vi "TcA02-009_TimeoutWhenWaitingForModifyingAttributes.vi"(1 "Input buffer":T3="1", 3 "Invocation info":T2, 5 "error in (no error)":errorcluster, 6 "Add log to result?":bool) -> (16 "Test Data":T1 {"Numeric Measurement" format="%.2f"}, 19 "error out":errorcluster)   [LabVIEW 2020]
doc: "Test case template."
uses:
  Shared/Support_InputBuffer.ctl
  Shared/Support_InvocationInfo.ctl
  Shared/Support_TestData.ctl
  TestClasses/G#BaseClass2_class/G#BaseClass2.lvclass
  TestClasses/G#SubClass2_class/G#SubClass2.lvclass
  TestClasses/G#SubSubClass2_class/G#SubSubClass2.lvclass
  <vilib>/addons/_AddQ/G#Object/G#Object.lvclass
panel:
  in  "Test name":string="TcA02-009 Timeout when waiting for modifying attributes"
  out "Test result":bool
  out "Result":string
  # "Verify that waiting for modifying objects attributes\nwhen mutual excluded can be timeout."
  # "Sub test case"
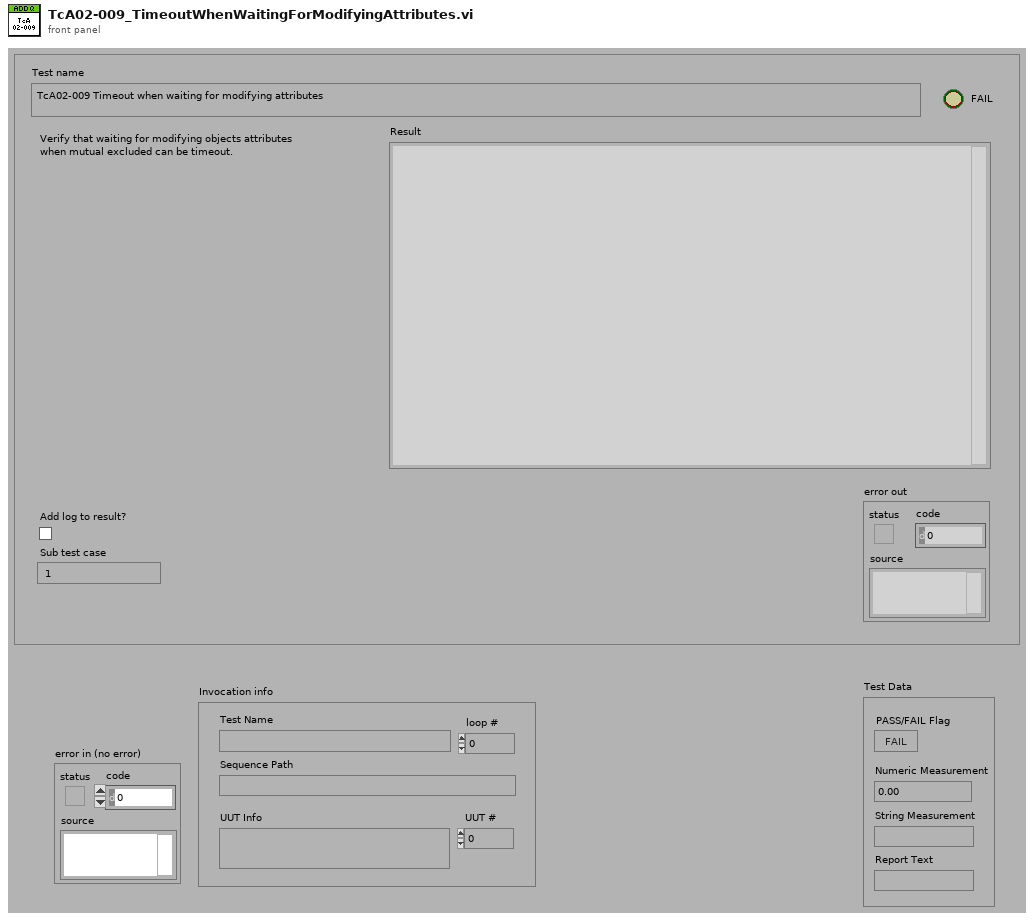
[diagram p1: front panel]
types:
  T1 = typedef "Support_TestData.ctl" = cluster{"PASS/FAIL Flag":bool, "Numeric Measurement":dbl, "String Measurement":string, "Report Text":string}
  T2 = typedef "Support_InvocationInfo.ctl" = cluster{"UUT #":i32, "loop #":i32, "UUT Info":string, "Test Name":string, "Sequence Path":path}
  T3 = typedef "Support_InputBuffer.ctl" = string
  T4 = typedef "Support_ResultType.ctl" = cluster{"Pass":bool, "Comment":string, "MeasurementValue":dbl}
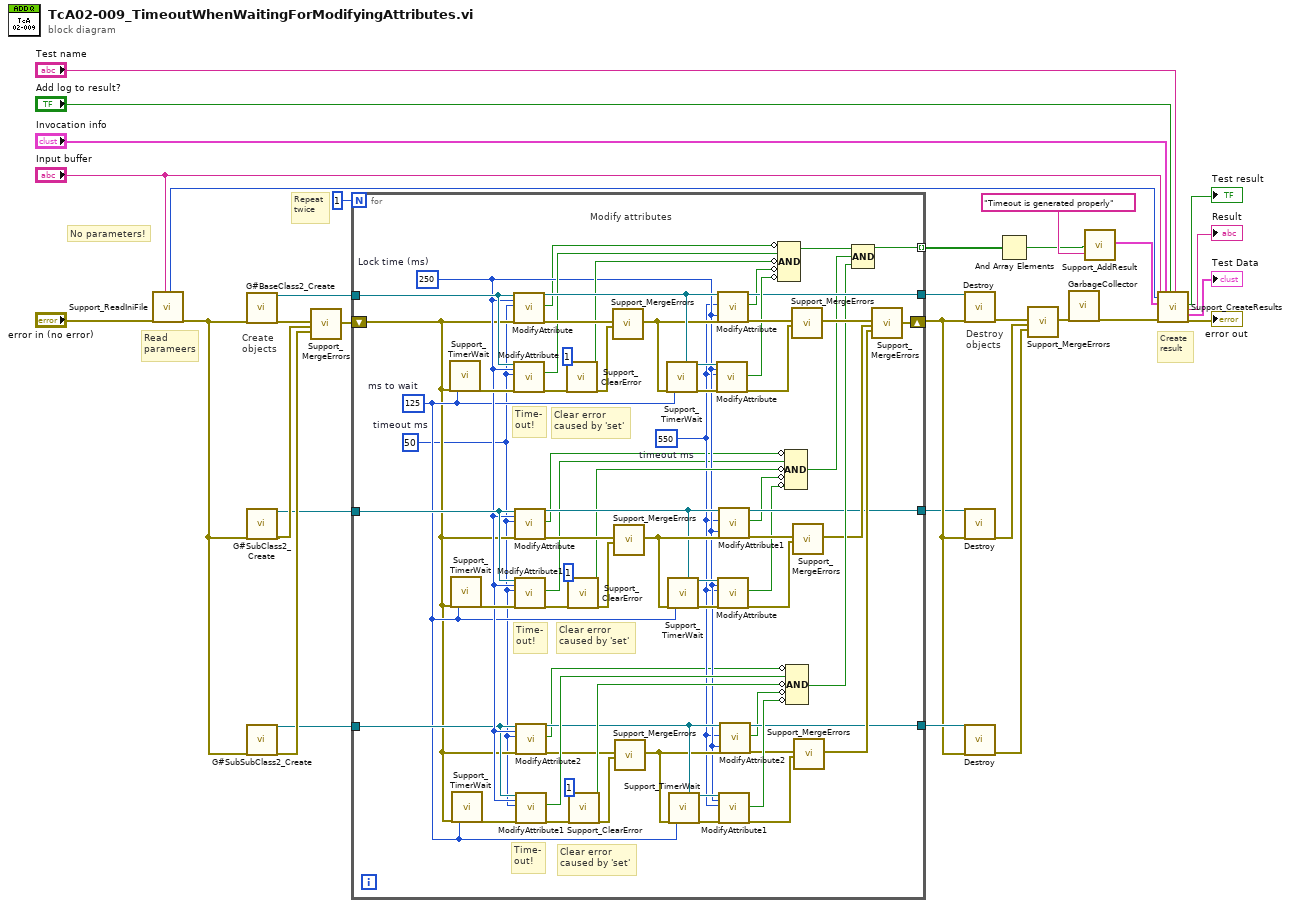
[diagram p0: block diagram]
diagram:
  # "Repeat\ntwice"
  # "Destroy\nobjects"
  # "Create\nobjects"
  # "No parameters!"
  # "Create\nresult"
  # "Read\nparameers"
  n1 = call "Support_ReadIniFile.vi"("error in (no error)"="error in (no error)", "Sub test case"="Input buffer") -> ("Timer start"=w23:u32, "error out"=w18:errorcluster)  [unwired: 10 in, 6 out]
  n2 = call "G#BaseClass2_Create.vi"("error in (no error)"=w18) -> ("reference out"=w11:refnum<class "G#BaseClass2.lvclass">, "error out"=w17:errorcluster)  [unwired: 17 in]
  n3 = call "G#SubClass2_Create.vi"("error in (no error)"=w18) -> ("reference out"=w9:refnum<class "G#SubClass2.lvclass">, "error out"=w16:errorcluster)  [unwired: 17 in]
  n4 = call "G#SubSubClass2_Create.vi"("error in (no error)"=w18) -> ("reference out"=w8:refnum<class "G#SubSubClass2.lvclass">, "error out"=w15:errorcluster)  [unwired: 17 in]
  n5 = call "Support_MergeErrors.vi"("error in 1"=w17, "error in 2"=w16, "error in 3"=w15) -> ("error out"=w5:errorcluster)  [unwired: 15 in, 1 out]
  n6 = for {
    N: 1 -> [_]
    tunnel: w11 -> [w94]
    tunnel: [w85] -> w10
    tunnel: w9 -> [w70]
    tunnel: [w66] -> w4 mode=indexing
    tunnel: w8 -> [w48]
    tunnel: [w47] -> w7
    shift-right: [w45] -> w6
    shift-left: w5 -> [w44]
    tunnel: [w43] -> w1
    w41 = 550  # timeout ms
    w42 = 50  # timeout ms
    w52 = u32 250  # Lock time (ms)
    w46 = u32 125  # ms to wait
    # "Time-\nout!"
    # "Time-\nout!"
    # "Time-\nout!"
    # "Clear error\ncaused by 'set'"
    # "Clear error\ncaused by 'set'"
    # "Clear error\ncaused by 'set'"
    # "Modify attributes"
    n7 = call "Support_TimerWait.vi"("error in (no error)"=w44, "milliseconds to wait"=w46) -> ("error out"=w95:errorcluster)  [unwired: 17 in]
    n8 = call "Support_TimerWait.vi"("error in (no error)"=w44, "milliseconds to wait"=w46) -> ("error out"=w72:errorcluster)  [unwired: 17 in]
    n9 = call "Support_TimerWait.vi"("error in (no error)"=w44, "milliseconds to wait"=w46) -> ("error out"=w61:errorcluster)  [unwired: 17 in]
    n10 = call-dynamic "ModifyAttribute.vi"("reference in"=w94, "Lock time (ms)"=w52, "timeout in ms (-1)"=w42, "error in (no error)"=w44) -> ("reference out"=w93:refnum<class "G#BaseClass2.lvclass">, "timeout"=w40:bool, "error out"=w96:errorcluster)  [unwired: 13 in]
    n11 = call-dynamic "ModifyAttribute.vi"("reference in"=w94, "Lock time (ms)"=w52, "timeout in ms (-1)"=w42, "error in (no error)"=w95) -> ("timeout"=w87:bool, "error out"=w84:errorcluster)  [unwired: 13 in, 1 out]
    n12 = call-dynamic "ModifyAttribute.vi"("reference in"=w70, "Lock time (ms)"=w52, "timeout in ms (-1)"=w42, "error in (no error)"=w44) -> ("reference out"=w73:refnum<class "G#SubClass2.lvclass">, "timeout"=w38:bool, "error out"=w71:errorcluster)  [unwired: 13 in]
    n13 = call-dynamic "ModifyAttribute1.vi"("reference in"=w70, "Lock time (ms)"=w52, "timeout in ms (-1)"=w42, "error in (no error)"=w72) -> ("timeout"=w37:bool, "error out"=w78:errorcluster)  [unwired: 13 in, 1 out]
    n14 = call-dynamic "ModifyAttribute2.vi"("reference in"=w48, "Lock time (ms)"=w52, "timeout in ms (-1)"=w42, "error in (no error)"=w44) -> ("reference out"=w60:refnum<class "G#SubSubClass2.lvclass">, "timeout"=w34:bool, "error out"=w62:errorcluster)  [unwired: 13 in]
    n15 = call-dynamic "ModifyAttribute1.vi"("reference in"=w48, "Lock time (ms)"=w52, "timeout in ms (-1)"=w42, "error in (no error)"=w61) -> ("timeout"=w65:bool, "error out"=w55:errorcluster)  [unwired: 13 in, 1 out]
    n16 = call "Support_ClearError.vi"("code"=1, "error in (no error)"=w84) -> ("Cleared?"=w81:bool, "error out"=w83:errorcluster)  [unwired: 16 in]
    n17 = call "Support_ClearError.vi"("code"=1, "error in (no error)"=w78) -> ("Cleared?"=w69:bool, "error out"=w79:errorcluster)  [unwired: 16 in]
    n18 = call "Support_ClearError.vi"("code"=1, "error in (no error)"=w55) -> ("Cleared?"=w63:bool, "error out"=w54:errorcluster)  [unwired: 16 in]
    n19 = call "Support_MergeErrors.vi"("error in 1"=w96, "error in 2"=w83) -> ("error out"=w88:errorcluster)  [unwired: 16 in, 1 out]
    n20 = call "Support_MergeErrors.vi"("error in 1"=w71, "error in 2"=w79) -> ("error out"=w77:errorcluster)  [unwired: 16 in, 1 out]
    n21 = call "Support_MergeErrors.vi"("error in 1"=w62, "error in 2"=w54) -> ("error out"=w56:errorcluster)  [unwired: 16 in, 1 out]
    n22 = call "Support_TimerWait.vi"("error in (no error)"=w88, "milliseconds to wait"=w46) -> ("error out"=w90:errorcluster)  [unwired: 17 in]
    n23 = call "Support_TimerWait.vi"("error in (no error)"=w77, "milliseconds to wait"=w46) -> ("error out"=w76:errorcluster)  [unwired: 17 in]
    n24 = call "Support_TimerWait.vi"("error in (no error)"=w56, "milliseconds to wait"=w46) -> ("error out"=w57:errorcluster)  [unwired: 17 in]
    n25 = call-dynamic "ModifyAttribute.vi"("reference in"=w93, "Lock time (ms)"=w52, "timeout in ms (-1)"=w41, "error in (no error)"=w90) -> ("timeout"=w86:bool, "error out"=w91:errorcluster)  [unwired: 13 in, 1 out]
    n26 = call-dynamic "ModifyAttribute.vi"("reference in"=w93, "Lock time (ms)"=w52, "timeout in ms (-1)"=w41, "error in (no error)"=w88) -> ("reference out"=w85:refnum<class "G#BaseClass2.lvclass">, "timeout"=w39:bool, "error out"=w92:errorcluster)  [unwired: 13 in]
    n27 = call-dynamic "ModifyAttribute.vi"("reference in"=w73, "Lock time (ms)"=w52, "timeout in ms (-1)"=w41, "error in (no error)"=w76) -> ("timeout"=w36:bool, "error out"=w75:errorcluster)  [unwired: 13 in, 1 out]
    n28 = call-dynamic "ModifyAttribute1.vi"("reference in"=w73, "Lock time (ms)"=w52, "timeout in ms (-1)"=w41, "error in (no error)"=w77) -> ("reference out"=w43:refnum<class "G#SubClass2.lvclass">, "timeout"=w35:bool, "error out"=w74:errorcluster)  [unwired: 13 in]
    n29 = call-dynamic "ModifyAttribute1.vi"("reference in"=w60, "Lock time (ms)"=w52, "timeout in ms (-1)"=w41, "error in (no error)"=w57) -> ("timeout"=w64:bool, "error out"=w58:errorcluster)  [unwired: 13 in, 1 out]
    n30 = call-dynamic "ModifyAttribute2.vi"("reference in"=w60, "Lock time (ms)"=w52, "timeout in ms (-1)"=w41, "error in (no error)"=w56) -> ("reference out"=w47:refnum<class "G#SubSubClass2.lvclass">, "timeout"=w33:bool, "error out"=w59:errorcluster)  [unwired: 13 in]
    n31 = Compound Arithmetic op=AND(invert w40, w87, invert w81, invert w39, invert w86) -> (w68:bool)
    n32 = Compound Arithmetic op=AND(invert w38, w37, invert w69, invert w35, invert w36) -> (w67:bool)
    n33 = Compound Arithmetic op=AND(invert w34, w65, invert w63, invert w33, invert w64) -> (w51:bool)
    n34 = call "Support_MergeErrors.vi"("error in 1"=w92, "error in 2"=w91) -> ("error out"=w89:errorcluster)  [unwired: 16 in, 1 out]
    n35 = call "Support_MergeErrors.vi"("error in 1"=w74, "error in 2"=w75) -> ("error out"=w50:errorcluster)  [unwired: 16 in, 1 out]
    n36 = call "Support_MergeErrors.vi"("error in 1"=w59, "error in 2"=w58) -> ("error out"=w49:errorcluster)  [unwired: 16 in, 1 out]
    n37 = Compound Arithmetic op=AND(w68, w67, w51) -> (w66:bool)
    n38 = call "Support_MergeErrors.vi"("error in 1"=w89, "error in 2"=w50, "error in 3"=w49) -> ("error out"=w45:errorcluster)  [unwired: 15 in, 1 out]
  }
  n39 = call-dynamic "Destroy.vi"("reference in"=w10, "error in (no error)"=w6) -> ("error out"=w14:errorcluster)  [unwired: 16 in, 1 out]
  n40 = call-dynamic "Destroy.vi"("reference in"=w1, "error in (no error)"=w6) -> ("error out"=w13:errorcluster)  [unwired: 16 in, 1 out]
  n41 = call-dynamic "Destroy.vi"("reference in"=w7, "error in (no error)"=w6) -> ("error out"=w12:errorcluster)  [unwired: 16 in, 1 out]
  n42 = And Array Elements(Boolean array=w4) -> (logical AND=w3:bool)
  n43 = call "Support_MergeErrors.vi"("error in 1"=w14, "error in 2"=w13, "error in 3"=w12) -> ("error out"=w22:errorcluster)  [unwired: 15 in, 1 out]
  n44 = call <vilib>:"GarbageCollector.vi"("error in (no error)"=w22) -> ("error out"=w21:errorcluster)  [unwired: 16 in, 2 out]
  n45 = call "Support_AddResult.vi"("Pass"=w3, "Comment"="Timeout is generated properly") -> ("Results out"=w20:T4[])  [unwired: 17 in]
  n46 = call "Support_CreateResults.vi"("Sub test case"="Input buffer", "Timer start"=w23, "Results"=w20, "error in (no error)"=w21, "Invocation info"="Invocation info", "Add log to result?"="Add log to result?", "Test name"="Test name") -> ("Pass/fail flag"=→"Test result":bool, "Result"=→"Result":string, "Test Data"=→"Test Data":T1, "error out"=→"error out":errorcluster)  [unwired: 9 in]
